vi "PathPlanner_PathFinder_New.vi"(8 "error in (no error)":errorcluster, 11 "NavGridFileName":string="default_navgrid.json") -> (0 "error out":errorcluster)   [LabVIEW 2019, in "PathPlanner24.lvlib"]
doc: "Create and initialize all data structures and back end VI (threads) needed by the Path Finder / Path Finding functions. Only one instance of this can be used at a time."
uses:
  PathPlanner24.lvlib
  TypeDef/PathPlannerFinderGridPosition.ctl
  ENum/PathPlanner_PathFinding_Cmd_ENUM.ctl
  9f52653c-7fec-4a5d-b71e-99ae675dab0e.vi
  PathPlanner_PathFinder_Globals.vi
  <vilib>/Rock Robotics/WPI/ThirdParty/JAS_Junk/TrajLib/Trajectory_Library.lvlib
panel:
  # "PURPOSEFULLY NON-REENTRANT"
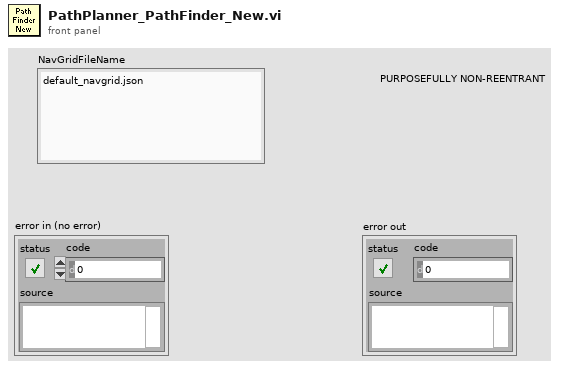
[diagram p1: front panel]
types:
  T1 = typedef "PathPlanner24.lvlib/PathPlanner_PathFinding_Cmd_ENUM.ctl" = enum16{"Do Nothing", "Reset", "Minor", "Reset and Minor", "Major", "Reset and Major", "Minor and Major", "Reset, Minor, Major"}
  T2 = typedef "PathPlanner24.lvlib/PathPlannerFinderGridPosition.ctl" = cluster{"X":i32, "Y":i32}
  T3 = typedef "PathPlanner24.lvlib/PathPlannerObstacleGrid.ctl" = cluster{"NodeSizeMeters":dbl, "Grid":bool[][], "NodeCountX":i32, "NodeCountY":i32, "FieldSizeX_M":dbl, "FieldSizeY_M":dbl}
  T4 = typedef "Trajectory_Library.lvlib/TRANSLATION2D.ctl" = cluster{"X":dbl, "Y":dbl}
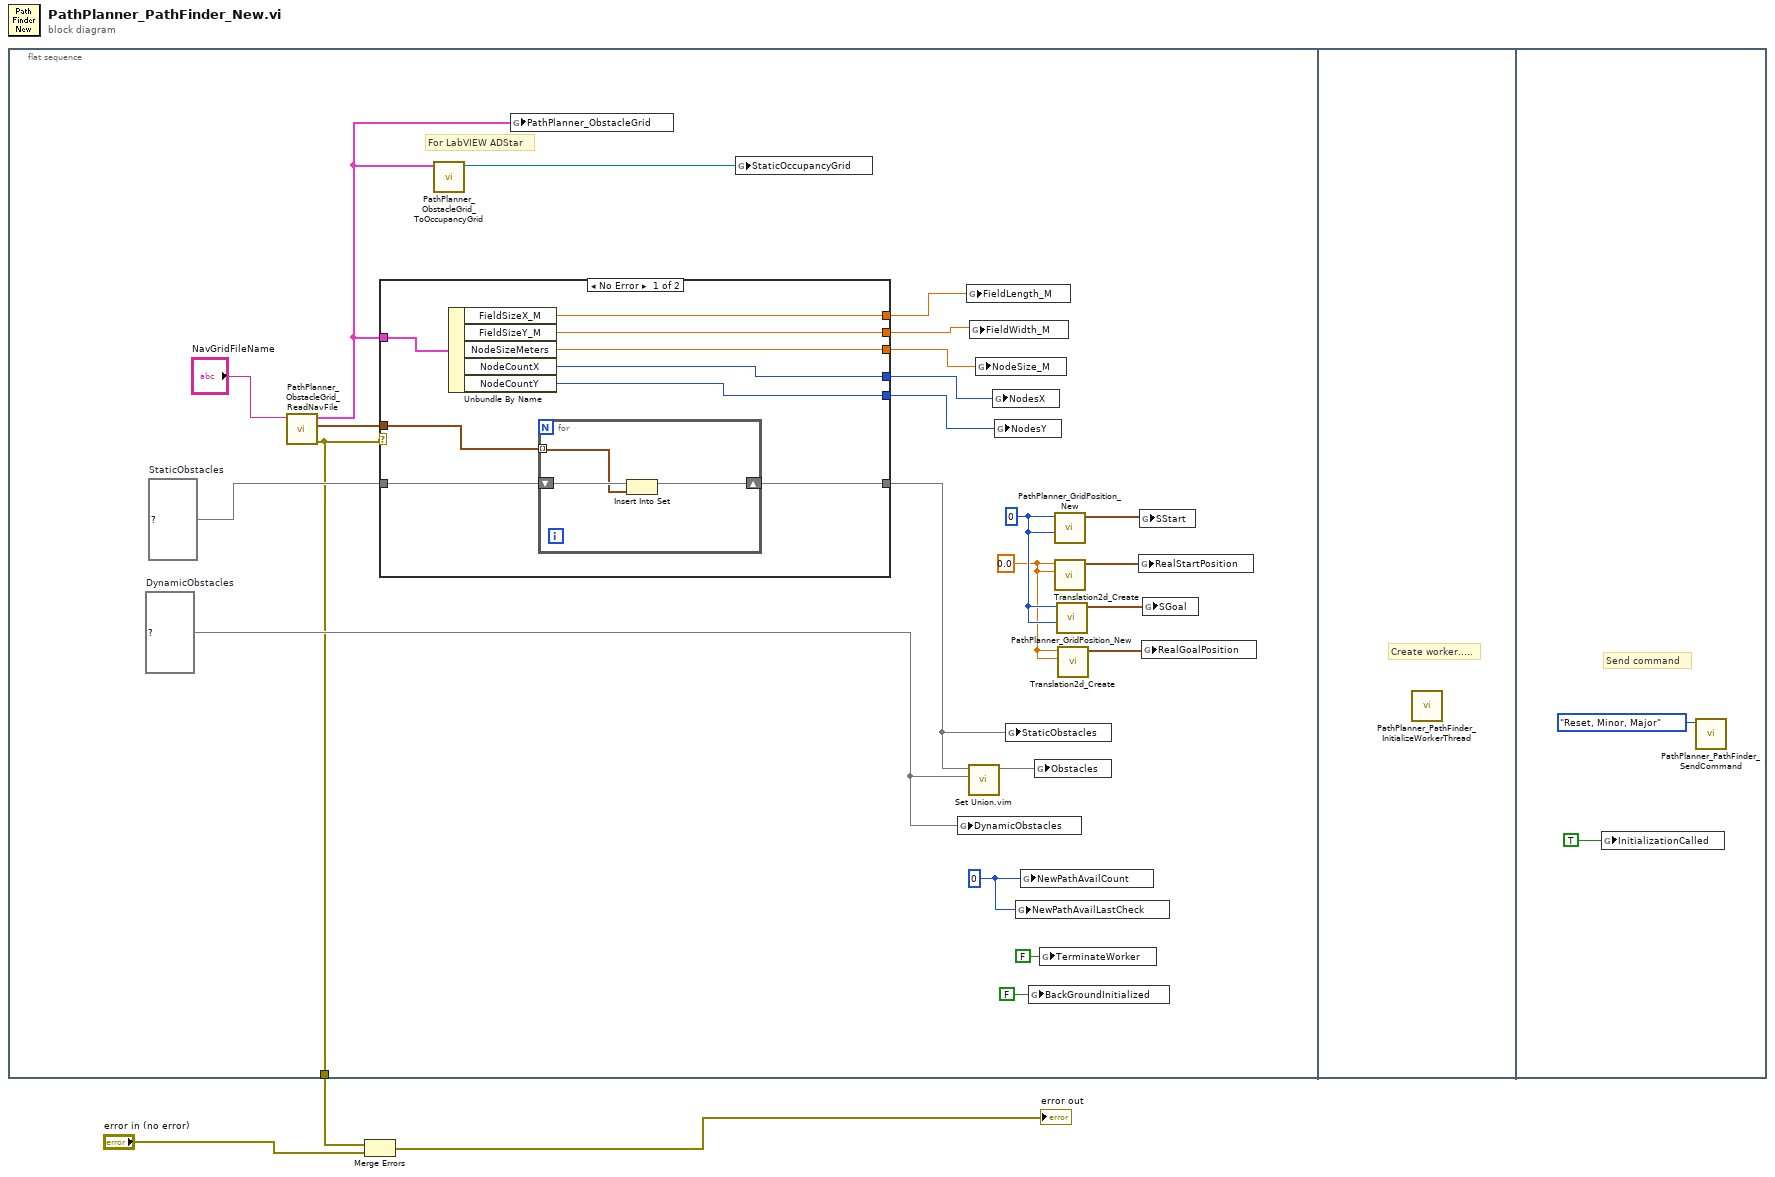
[diagram p0: block diagram]
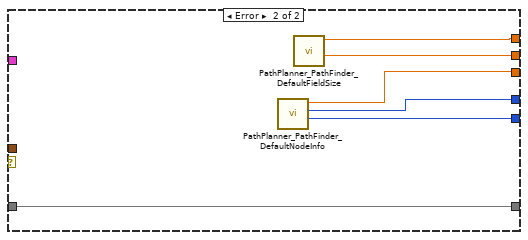
[diagram p2: hidden frame]
diagram:
  n1 = flat-sequence {
    tunnel: [w7] -> w3
    frame #0 {
      w8 = set{T2} {}  # DynamicObstacles
      w11 = set{T2} {}  # StaticObstacles
      w12 = 0 ("NewPathAvailCount")
      w18 = 0.0 ("X")
      w19 = 0 ("X")
      # "For LabVIEW ADStar"
      n2 = call "PathPlanner_ObstacleGrid_ReadNavFile.vi"("FileName"="NavGridFileName") -> ("error out"=w7:errorcluster, "NavGridObstacles"=w20:T2[], "PathPlanner_Grid"=w4:T3)  [unwired: 7 in, 1 out]
      n3 = case shown="No Error" w7 {
        tunnel: w4 -> [w35 _]
        tunnel: [w34 w44] -> w25
        tunnel: [w33 w43] -> w24
        tunnel: [w32 w42] -> w23
        tunnel: [w31 w41] -> w22
        tunnel: [w30 w40] -> w21
        tunnel: w20 -> [w29 _]
        tunnel: w11 -> [w28 w39]
        tunnel: [w27 w39] -> w9
        frame No Error {
          n4 = Unbundle By Name(w35) -> ("FieldSizeX_M"=w34:dbl, "FieldSizeY_M"=w33:dbl, "NodeSizeMeters"=w32:dbl, "NodeCountX"=w31:i32, "NodeCountY"=w30:i32)
          n5 = for {
            tunnel: w29 -> [w36] mode=indexing
            shift-right: [w37] -> w27
            shift-left: w28 -> [w38]
            n6 = Insert Into Set(10:w36, 11:w38) -> (3:w37:set{T2})  [unwired: 1 out]
          }
        }
        frame Error {
          n7 = call "PathPlanner_PathFinder_DefaultNodeInfo.vi"() -> ("fieldWidth_Meters"=w40:i32, "fieldLength_Meters"=w41:i32, "NodeSize_Meters"=w42:dbl)  [unwired: 9 in]
          n8 = call "PathPlanner_PathFinder_DefaultFieldSize.vi"() -> ("fieldWidth_Meters"=w43:dbl, "fieldLength_Meters"=w44:dbl)  [unwired: 10 in]
        }
      }
      n9 = call "PathPlanner_ObstacleGrid_ToOccupancyGrid.vi"("PathPlanner_Grid"=w4) -> ("map reference out"=w13:refnum<data-value>)  [unwired: 9 in, 1 out]
      n10 = global write "PathPlanner_PathFinder_Globals.vi" "PathPlanner_ObstacleGrid"(w4) -> ()
      n11 = global write "PathPlanner_PathFinder_Globals.vi" "StaticOccupancyGrid"(w13) -> ()
      n12 = global write "PathPlanner_PathFinder_Globals.vi" "DynamicObstacles"(w8) -> ()
      n13 = global write "PathPlanner_PathFinder_Globals.vi" "FieldLength_M"(w25) -> ()
      n14 = call "Set Union.vim"("set 2"=w8, "set 1"=w9) -> ("union"=w10:set{T2})  [unwired: 9 in]
      n15 = global write "PathPlanner_PathFinder_Globals.vi" "FieldWidth_M"(w24) -> ()
      n16 = global write "PathPlanner_PathFinder_Globals.vi" "NodeSize_M"(w23) -> ()
      n17 = global write "PathPlanner_PathFinder_Globals.vi" "NodesX"(w22) -> ()
      n18 = global write "PathPlanner_PathFinder_Globals.vi" "NodesY"(w21) -> ()
      n19 = global write "PathPlanner_PathFinder_Globals.vi" "StaticObstacles"(w9) -> ()
      n20 = global write "PathPlanner_PathFinder_Globals.vi" "NewPathAvailLastCheck"(w12) -> ()
      n21 = global write "PathPlanner_PathFinder_Globals.vi" "NewPathAvailCount"(w12) -> ()
      n22 = global write "PathPlanner_PathFinder_Globals.vi" "BackGroundInitialized"(FALSE ("TerminateWorker")) -> ()
      n23 = global write "PathPlanner_PathFinder_Globals.vi" "Obstacles"(w10) -> ()
      n24 = global write "PathPlanner_PathFinder_Globals.vi" "TerminateWorker"(FALSE ("TerminateWorker")) -> ()
      n25 = call "PathPlanner_GridPosition_New.vi"("Int Y"=w19, "Int X"=w19) -> ("GridPosition"=w17:T2)  [unwired: 9 in]
      n26 = call <vilib>:"Translation2d_Create.vi"("Y"=w18, "X"=w18) -> ("TRANSLATION"=w16:T4)  [unwired: 9 in]
      n27 = call "PathPlanner_GridPosition_New.vi"("Int Y"=w19, "Int X"=w19) -> ("GridPosition"=w15:T2)  [unwired: 9 in]
      n28 = call <vilib>:"Translation2d_Create.vi"("Y"=w18, "X"=w18) -> ("TRANSLATION"=w14:T4)  [unwired: 9 in]
      n29 = global write "PathPlanner_PathFinder_Globals.vi" "RealStartPosition"(w16) -> ()
      n30 = global write "PathPlanner_PathFinder_Globals.vi" "SStart"(w17) -> ()
      n31 = global write "PathPlanner_PathFinder_Globals.vi" "RealGoalPosition"(w14) -> ()
      n32 = global write "PathPlanner_PathFinder_Globals.vi" "SGoal"(w15) -> ()
    }
    frame #1 {
      # "Create worker....."
      n33 = call "PathPlanner_PathFinder_InitializeWorkerThread.vi"() -> ()  [unwired: 12 in]
    }
    frame #2 {
      # "Send command"
      n34 = global write "PathPlanner_PathFinder_Globals.vi" "InitializationCalled"(TRUE ("TerminateWorker")) -> ()
      n35 = call "PathPlanner_PathFinder_SendCommand.vi"("PathFindingCommand"=PathPlanner_PathFinding_Cmd_ENUM."Reset, Minor, Major") -> ()  [unwired: 10 in, 1 out]
    }
  }
  n36 = Merge Errors(w3, "error in (no error)") -> (→"error out":errorcluster)
